vi "Add Tree Items.vi"(8 "error in (no error)":errorcluster, 9 "Actual Path":path[](array[path]), 10 "Expected Path":path[](array[path]), 11 "Tree Refnum":refnum<vi>) -> (0 "error out":errorcluster, 2 "Tree Map":map{path, T1}(c390), 3 "Tree Refnum out":refnum<vi>)   [LabVIEW 2023]
doc: "Populates the tree control identified by <B>Tree Refnum</B> with the other inputs."
uses:
  CTLs/Tree Map Value.ctl
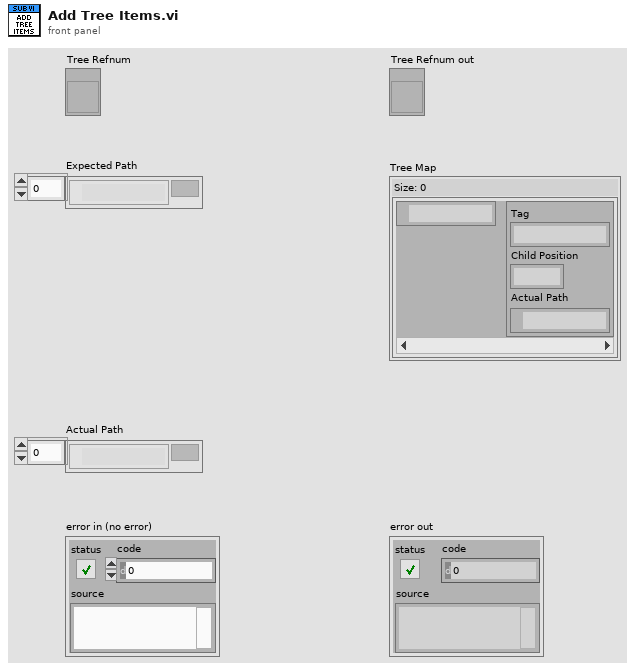
[diagram p1: front panel]
types:
  T1 = typedef "Tree Map Value.ctl" = cluster{"Tag":string, "Child Position":i32, "Actual Path":path}
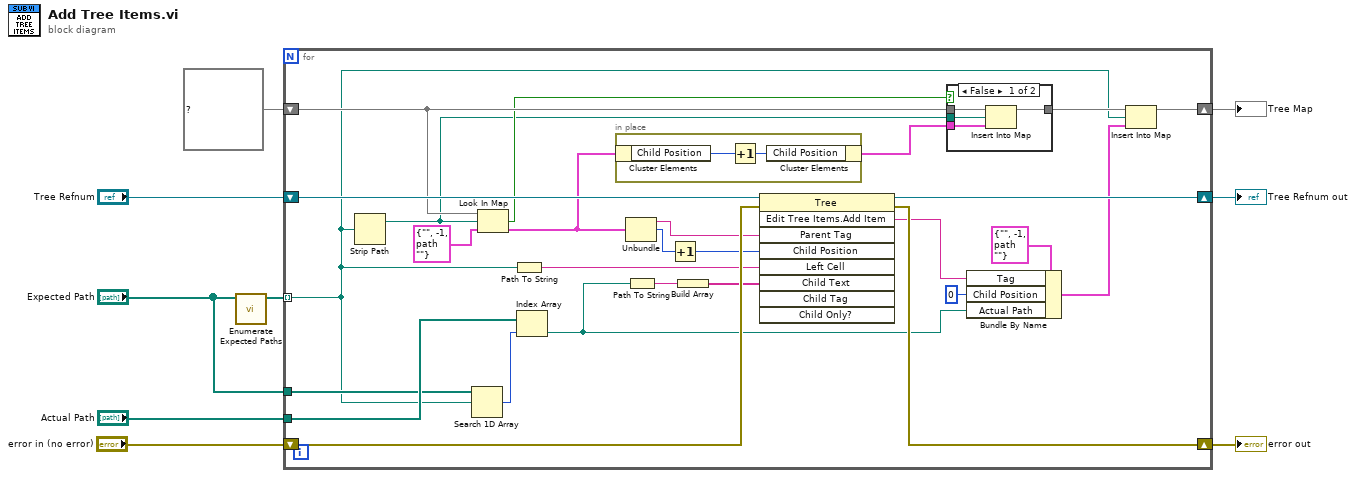
[diagram p0: block diagram]
diagram:
  n1 = call "Enumerate Expected Paths.vi"("Expected Path"="Expected Path") -> ("Enumerated Expected Paths"=w4:path[])  [unwired: 10 in]
  n2 = for {
    tunnel: w4 -> [w18] mode=indexing
    shift-right: [w17] -> w5
    shift-left: map{path, T1} {} ("map") -> [w26]
    shift-right: [w33] -> w7
    shift-left: "Tree Refnum" -> [w34]
    tunnel: "Actual Path" -> [w32]
    tunnel: "Expected Path" -> [w31]
    shift-right: [w35] -> w1
    shift-left: "error in (no error)" -> [w36]
    n3 = Strip Path(path=w18) -> (stripped path=w19:path)  [unwired: 1 out]
    n4 = Search 1D Array(1D array=w31, element=w18) -> (index of element=w27:i32)  [unwired: 1 in]
    n5 = Look In Map(map=w26, key=w19, default value=T1 {"Tag"="", "Child Position"=-1, "Actual Path"=path ""}) -> (key not found?=w20:bool, value=w11:T1)
    n6 = Path To String(path=w18) -> (string=w29:string)
    n7 = Index Array(array=w32, index=w27) -> (element=w13:path)
    n8 = in-place {
      n9 = in-place-cluster #1(w11) -> ("Child Position"=w38:i32)
      n10 = Increment(x=w38) -> (x+1=w37:i32)
      n11 = in-place-cluster #1("Child Position"=w37) -> (w10:T1)
    }
    n12 = Unbundle(w11) -> ("Tag"=w22:string, "Child Position"=w23:i32)  [unwired: 1 out]
    n13 = Path To String(path=w13) -> (string=w28:string)
    n14 = Increment(x=w23) -> (x+1=w21:i32)
    n15 = Build Array(w28) -> (w30:string[])
    n16 = invoke class="Tree" method="Edit Tree Items.Add Item"(reference=w34, error in=w36, "Parent Tag"=w22, "Child Position"=w21, "Left Cell"=w29, "Child Text"=w30) -> (reference out=w33:refnum<vi>, error out=w35:errorcluster, "Edit Tree Items:Add Item"=w15:string)  [unwired: 3 in, 6 out]
    n17 = case shown="False" w20 {
      tunnel: w26 -> [w42 w43]
      tunnel: [w41 w43] -> w25
      tunnel: w10 -> [w40 _]
      tunnel: w19 -> [w39 _]
      frame False {
        n18 = Insert Into Map(map in=w42, key=w39, value=w40) -> (map out=w41:map{path, T1})  [unwired: 2 out]
      }
      frame True {
      }
    }
    n19 = Bundle By Name(cluster=T1 {"Tag"="", "Child Position"=-1, "Actual Path"=path ""} ("default value"), "Tag"=w15, "Child Position"=0, "Actual Path"=w13) -> (w12:T1)
    n20 = Insert Into Map(map in=w25, key=w18, value=w12) -> (map out=w17:map{path, T1})  [unwired: 2 out]
  }
  "Tree Refnum out" <- w7
  "Tree Map" <- w5
  "error out" <- w1
